vi "Measurement tester.vi"() -> ()   [LabVIEW 2016]
uses:
  Modulation_Signals.ctl
panel:
  in  "Input channels":cluster{string, "physical channels":tag}[](array[cluster])
  out "Waveform Graph":waveform(dbl)[](graph)
  in  "Frequency 2":dbl
  in  "Samples":dbl format="%#_13g"
  in  "Signal Type":T1
  in  "Frequency 1":dbl
  in  "Sampling rate":dbl format="%#_13g"
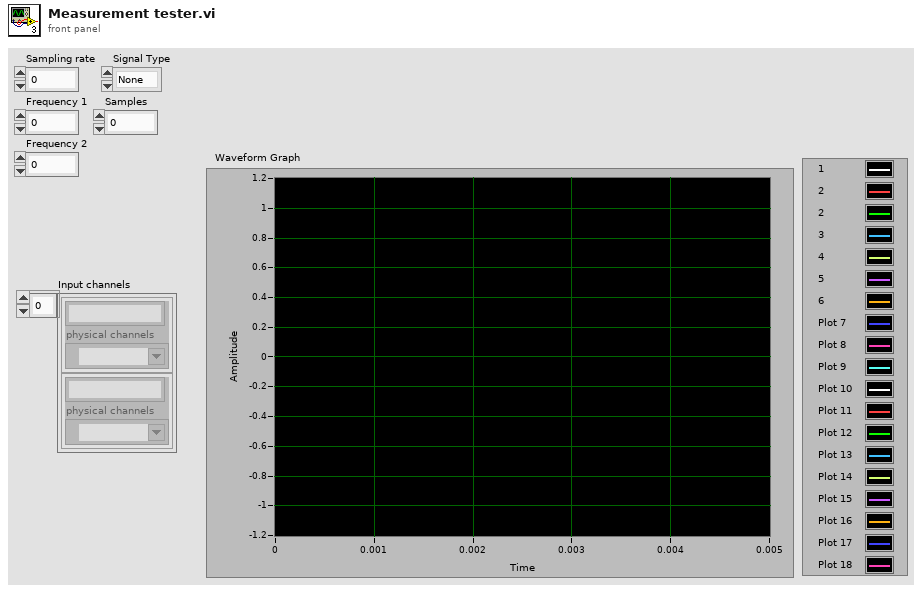
[diagram p1: front panel]
types:
  T1 = typedef "Modulation_Signals.ctl" = enum16{"None", "Sine", "Chirp", "White Noise", "File"}
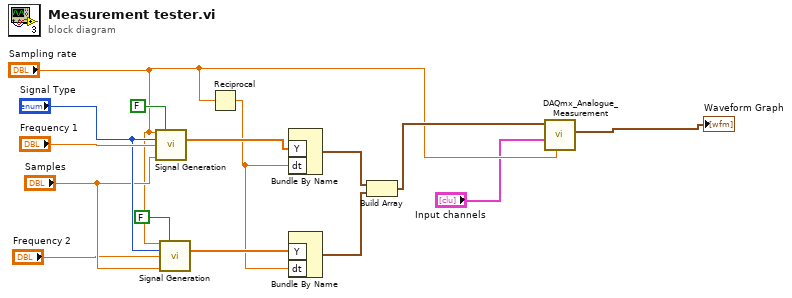
[diagram p0: block diagram]
diagram:
  n1 = call "Signal Generation.vi"("Output Fs"="Sampling rate", "Filter"=FALSE, "Signal Type"="Signal Type", "Frequency 1"="Frequency 1", "Samples"="Samples") -> ("Output Signal"=w8:dbl[])  [unwired: 10 in]
  n2 = call "Signal Generation.vi"("Output Fs"="Sampling rate", "Filter"=FALSE, "Signal Type"="Signal Type", "Frequency 1"="Frequency 2", "Samples"="Samples") -> ("Output Signal"=w9:dbl[])  [unwired: 10 in]
  n3 = Reciprocal(x="Sampling rate") -> (1/x=w7:dbl)
  n4 = Bundle By Name("Y"=w8, "dt"=w7) -> (w6:waveform(dbl))  [unwired: 1 in]
  n5 = Bundle By Name("Y"=w9, "dt"=w7) -> (w5:waveform(dbl))  [unwired: 1 in]
  n6 = Build Array(w6, w5) -> (w3:waveform(dbl)[])
  n7 = call "DAQmx_Analogue_Measurement.vi"("Sampling rate"="Sampling rate", "Input channels"="Input channels", "Outputs"=w3) -> ("Measured data"=→"Waveform Graph":waveform(dbl)[])  [unwired: 7 in, 1 out]
